vi "AB_API Create Library For Destination.vi"(8 "error in (no error)":errorcluster, 9 "New project library name":string, 10 "Destination label":string, 11 "Build in":refnum<class "AB_Build.lvclass">) -> (0 "error out":errorcluster, 3 "Build out":refnum<class "AB_Build.lvclass">)   [LabVIEW 2020]
uses:
  <vilib>/AppBuilder/AB_Classes/Build/AB_Build.lvclass
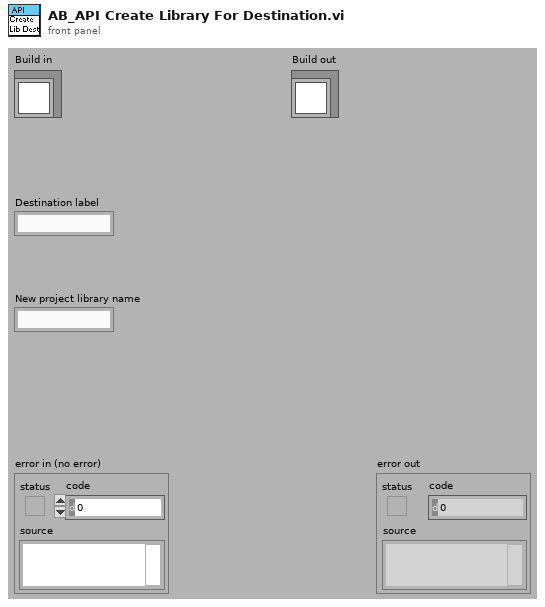
[diagram p1: front panel]
types:
  T1 = typedef "AB_Build.ctl" = cluster{"buildSpecName":string, "buildSpecDescription":string, "destinations":refnum<class "AB_Destination.lvclass">[], "exclusionOption":T2, "defaultLanguage":string, "supportedLanguages":string[], "excludedDirectories":path[], "buildContext":refnum<vi>, "buildObject":T3, "preview":bool, "programatic":bool, "progressBarEvents":T4, "userLog_Path":path, "preActionID":string, "preAction_Path":path, "postActionID":string, "postAction_Path":path, "eng_checkForBrokenVIs?":bool, "eng_verboseLinkerErrors?":bool, "localDest_Path":path, "targetDest_Path":path, "removeVIObject":u16, "cache":refnum<class "PreviewCache.lvclass">, "use cache":bool, "previewCache_ID":string, "buildCache_ID":string, "eng_TempLocalDest_Path":path, "eng_collectDependencies?":bool, "versionInfo":cluster{"buildVersion":cluster{"major":u16, "minor":u16, "patch":u16, "build":u16}, "autoIncrement":bool}, "eng_enableVIChecksums":bool}
  T2 = typedef "AB_Exclusion_Option.ctl" = cluster{"typedefs":bool, "polymorphicVIs":bool, "unusedLibraryItems":bool, "modifyLibraryFile":bool, "edit-timeDependencies":bool, "inlineVIs":bool, "dependent PPLs":bool, "dependent DLLs":bool}
  T3 = typedef "ItemRef.ctl" = u64
  T4 = typedef "provcom_ProgressBar_Events.ctl" = cluster{"newJob":refnum<user-event>, "newItem":refnum<user-event>, "errorMsg":T5, "cancel":refnum<user-event>}
  T5 = typedef "mxLvBuildError.ctl" = refnum<user-event>
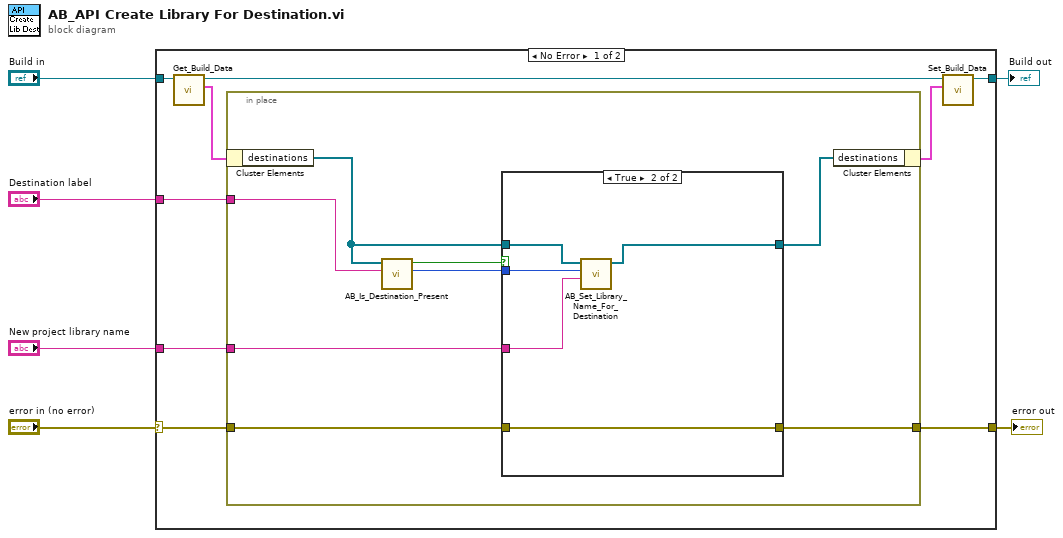
[diagram p0: block diagram]
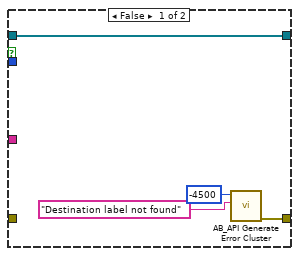
[diagram p2: hidden frame]
diagram:
  n1 = case shown="No Error" "error in (no error)" {
    selector: "error in (no error)" -> [w9 w34]
    tunnel: [w8 w34] -> w5
    tunnel: "Build in" -> [w12 w33]
    tunnel: [w11 w33] -> w3
    tunnel: "Destination label" -> [w10 _]
    tunnel: "New project library name" -> [w7 _]
    frame No Error {
      n2 = call <vilib>:"Get_Build_Data.vi"("Class in"=w12) -> ("data"=w14:T1, "Class out"=w15:refnum<class "AB_Build.lvclass">)  [unwired: 1 in, 8 out]
      n3 = in-place {
        in-place-border: w7 -> [w22]
        in-place-border: w10 -> [w16]
        in-place-border: [w21] -> w8
        in-place-border: w9 -> [w20]
        n4 = in-place-cluster #1(w14) -> ("destinations"=w19:refnum<class "AB_Destination.lvclass">[])
        n5 = call <vilib>:"AB_Is_Destination_Present.vi"("destination label"=w16, "destinations"=w19) -> ("index"=w18:i32, "destination present?"=w17:bool)  [unwired: 1 in, 7 out]
        n6 = case shown="True" w17 {
          tunnel: [w27 w30] -> w23
          tunnel: w22 -> [_ w28]
          tunnel: w19 -> [w27 w31]
          tunnel: w18 -> [_ w29]
          tunnel: [w25 w32] -> w21
          tunnel: w20 -> [_ w32]
          frame False {
            n7 = call <vilib>:"AB_API Generate Error Cluster.vi"("Additional Message"="Destination label not found", "Code"=-4500) -> ("error out"=w25:errorcluster)  [unwired: 2 in, 7 out]
          }
          frame True {
            n8 = call <vilib>:"AB_Set_Library_Name_For_Destination.vi"("library name"=w28, "destination index"=w29, "destinations in"=w31) -> ("destinations out"=w30:refnum<class "AB_Destination.lvclass">[])  [unwired: 2 in, 6 out]
          }
        }
        n9 = in-place-cluster #1("destinations"=w23) -> (w13:T1)
      }
      n10 = call <vilib>:"Set_Build_Data.vi"("data"=w13, "Class in"=w15) -> ("Class out"=w11:refnum<class "AB_Build.lvclass">)  [unwired: 1 in, 8 out]
    }
    frame Error {
    }
  }
  "error out" <- w5
  "Build out" <- w3
